vi "PosStrikerAnguloAttacker.vi"(8 "AnguloGol":dbl, 9 "atacando contra":bool, 10 "IA State":T1={"our_robots"=[], "enemy_robots"=[], "balls"=[], "geometry"={"line_width"=0, "field_length"=0, "field_width"=0, "boundary_width"=0, "referee_width"=0, "goal_width"=0, "goal_depth"=0, "goal_wall_width"=0, "center_circle_radius"=0, "defense_radius"=0, "defense_stretch"=0, "free_kick_from_defense_dist"=0, "penalty_spot_from_field_line_dist"=0, "penalty_line_from_spot_dist"=0}, "IA Judge"={"stage"="", "command"="", "our_goalie_id"=0.0, "enemy_goalie_id"=0.0, "command enum"=enum."Halt", "Time"=enum."Azul"}, "Received Timestamp"=timestamp(0 s since 1904-01-01), "Events"={"Touch"=FALSE, "Ball out"=FALSE, "id touch"=0.0, "Ball out of \nVision"=FALSE, "Ball inside \nGoalie area"=FALSE, "Robot not responding"=FALSE, "Robots responding status"=[1.0, 1.0, 1.0, 1.0, 1.0, 1.0], "Enemy Ball \nPossession"=FALSE, "Pass State"=FALSE, "id end of pass"=0.0, "Kick"=FALSE, "Id ini Possession"=0.0, "Ball Possesion"=FALSE, "Id Possesion"=0.0}}) -> (0 "YdoAttacker 2":dbl, 1 "AttackerPositive?":bool, 2 "theta final":dbl, 3 "XdoAttacker 2":dbl)   [LabVIEW 2017]
uses:
  Core/AI Input.ctl
  Core/AI Robot.ctl
  Intel/Functions Enum.ctl
  Intel/AttackerStates.ctl
  Core/AI Ball.ctl
  Core/Field Size.ctl
  Core/AI Judge.ctl
  Intel/Command Enum.ctl
  Events/Events.ctl
panel:
  in  "valor de theta 3":dbl
  in  "tamanho do intervalo 3":dbl
  in  "inicio do intervalo 3":dbl
  in  "fim do intervalo 3":dbl
  in  "Contador 4":dbl
  in  "Array 3":dbl[](array[numeric])=[0.0, 0.0, 0.0, 0.0, 0.0, 0.0]
  in  "valor de theta 2":dbl
  in  "tamanho do intervalo 2":dbl
  in  "inicio do intervalo 2":dbl
  in  "fim do intervalo 2":dbl
  in  "Contador 3":dbl
  in  "Array 2":dbl[](array[numeric])=[0.0, 0.0, 0.0, 0.0, 0.0, 0.0]
  in  "XdoAttacker":dbl
  in  "YdoAttacker":dbl
  in  "RobôsParaAnalisar":dbl[][](array[numeric])=[[99999.0, 99999.0], [99999.0, 99999.0], [99999.0, 99999.0], [99999.0, 99999.0], [99999.0, 99999.0], [99999.0, 99999.0], [99999.0, 99999.0]]
  in  "Contador":dbl
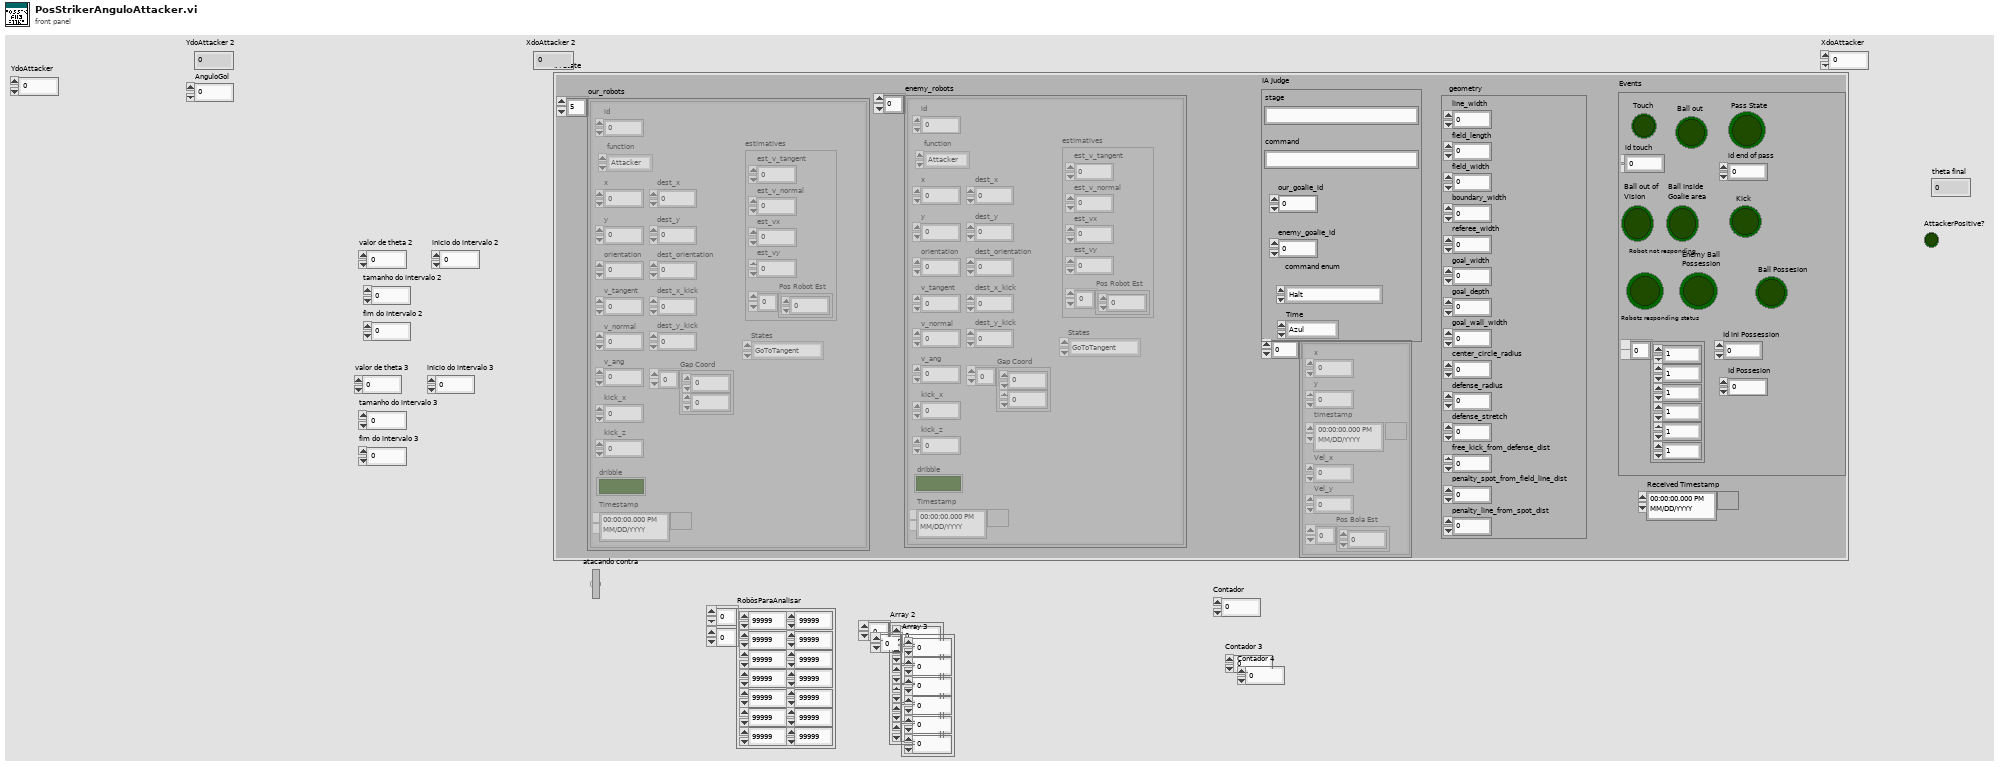
[diagram p1: front panel]
types:
  T1 = typedef "AI Input.ctl" = cluster{"our_robots":T2[], "enemy_robots":T2[], "balls":T5[], "geometry":T6, "IA Judge":T7, "Received Timestamp":timestamp, "Events":T9}
  T2 = typedef "AI Robot.ctl" = cluster{"id":u32, "function":T3, "x":dbl, "y":dbl, "orientation":dbl, "v_tangent":dbl, "v_normal":dbl, "v_ang":dbl, "kick_x":dbl, "kick_z":dbl, "dribble":bool, "Timestamp":timestamp, "dest_x":dbl, "dest_y":dbl, "dest_orientation":dbl, "estimatives":cluster{"est_v_tangent":dbl, "est_v_normal":dbl, "est_vx":dbl, "est_vy":dbl, "Pos Robot Est":dbl[]}, "dest_x_kick":dbl, "dest_y_kick":dbl, "Gap Coord":dbl[], "States":T4}
  T3 = typedef "Functions Enum.ctl" = enum16{"Attacker", "Goalie", "Defender", "Striker", "Goto 0", "Dummy", "Kicker", "ZigZag"}
  T4 = typedef "AttackerStates.ctl" = enum16{"Pass", "GoToTangent", "BallGetting", "GoToKick", ""}
  T5 = typedef "AI Ball.ctl" = cluster{"x":dbl, "y":dbl, "timestamp":timestamp, "Vel_x":dbl, "Vel_y":dbl, "Pos Bola Est":dbl[]}
  T6 = typedef "Field Size.ctl" = cluster{"line_width":u32, "field_length":u32, "field_width":u32, "boundary_width":u32, "referee_width":u32, "goal_width":u32, "goal_depth":u32, "goal_wall_width":u32, "center_circle_radius":u32, "defense_radius":u32, "defense_stretch":u32, "free_kick_from_defense_dist":u32, "penalty_spot_from_field_line_dist":u32, "penalty_line_from_spot_dist":u32}
  T7 = typedef "AI Judge.ctl" = cluster{"stage":string, "command":string, "our_goalie_id":dbl, "enemy_goalie_id":dbl, "command enum":T8, "Time":enum16{"Azul", "Amarelo"}}
  T8 = typedef "Command Enum.ctl" = enum16{"Halt", "Stop", "Force Start", "PKA Normal Start", "Prepare Kickoff Ally", "PKE Normal Start", "Prepare Kickoff Enemy", "Prepare Penalty Ally", "PPA Normal Start", "Prepare Penalty Enemy", "PPE Normal Start", "Direct Free Enemy", "Direct Free Ally", "Indirect Free Enemy", "Indirect Free Ally", "Timeout Enemy", "Timeout Ally", "Goal Enemy", "Goal Ally", "Ball Placement Enemy", "Ball Placement Ally", "Normal Half Time", "Extra Time Break", "Extra Half Time", "None", "Post Game"}
  T9 = typedef "Events.ctl" = cluster{"Touch":bool, "Ball out":bool, "id touch":dbl, "Ball out of \nVision":bool, "Ball inside \nGoalie area":bool, "Robot not responding":bool, "Robots responding status":dbl[], "Enemy Ball \nPossession":bool, "Pass State":bool, "id end of pass":dbl, "Kick":bool, "Id ini Possession":dbl, "Ball Possesion":bool, "Id Possesion":dbl}
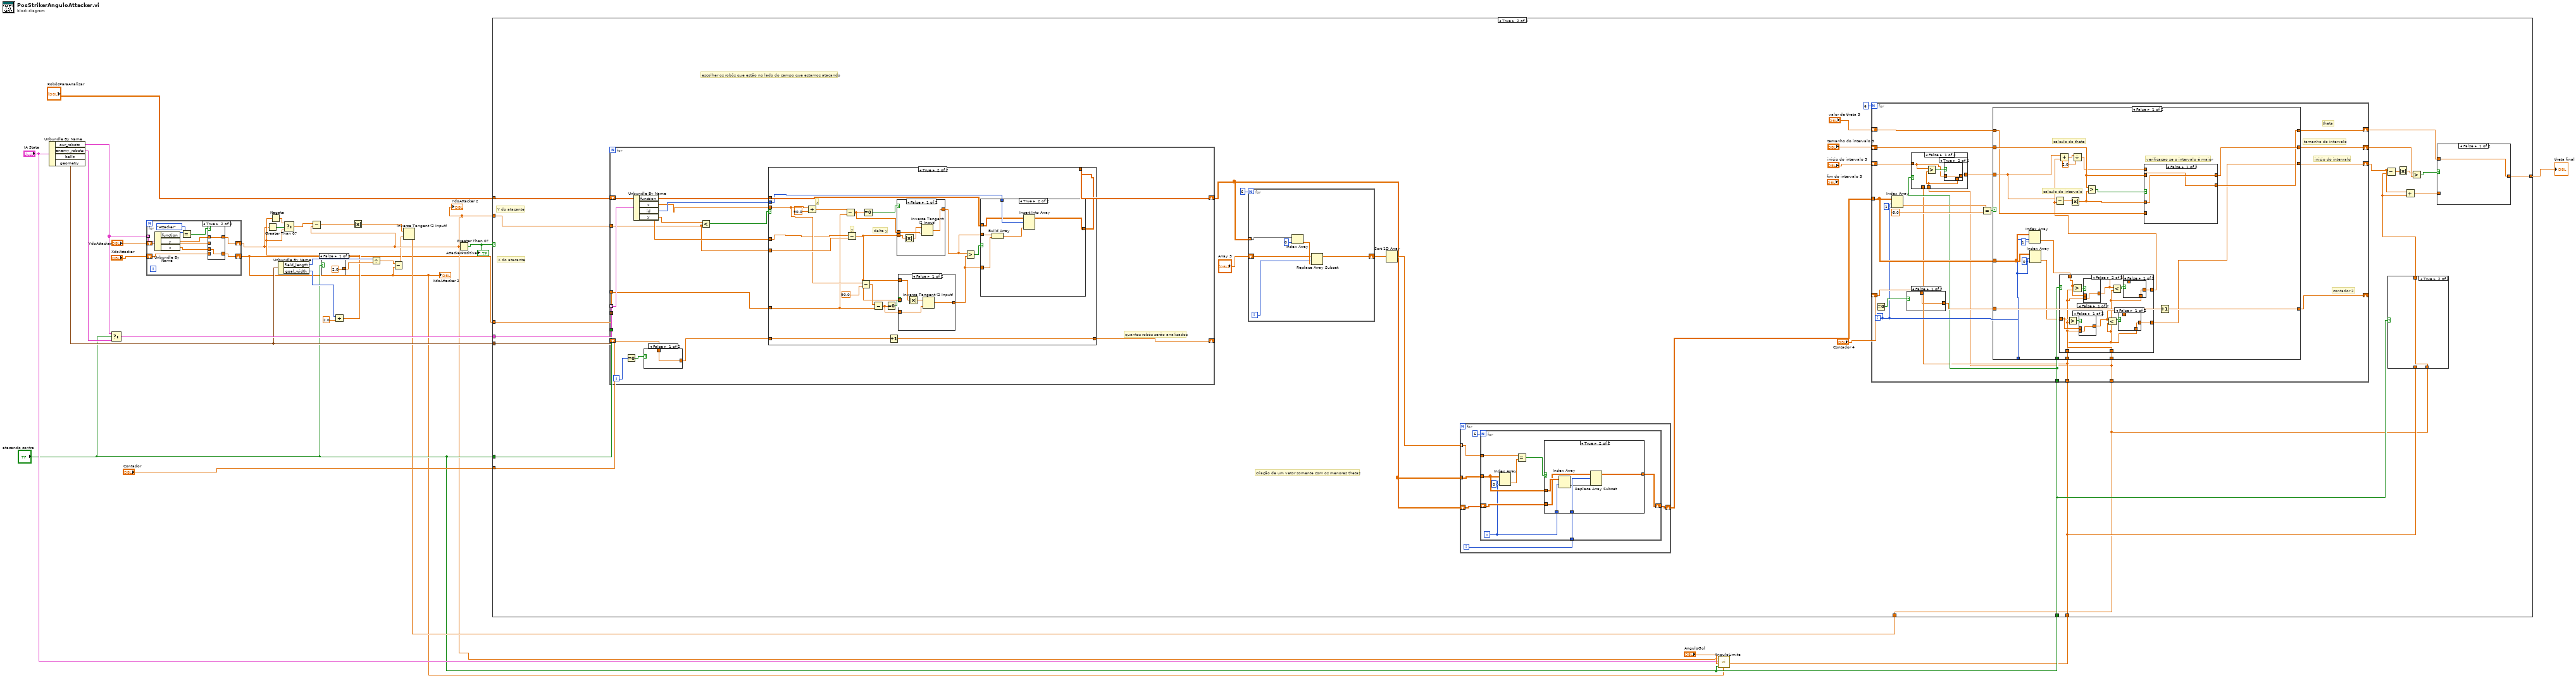
[diagram p0: block diagram]
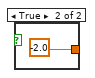
[diagram p2: hidden frame]
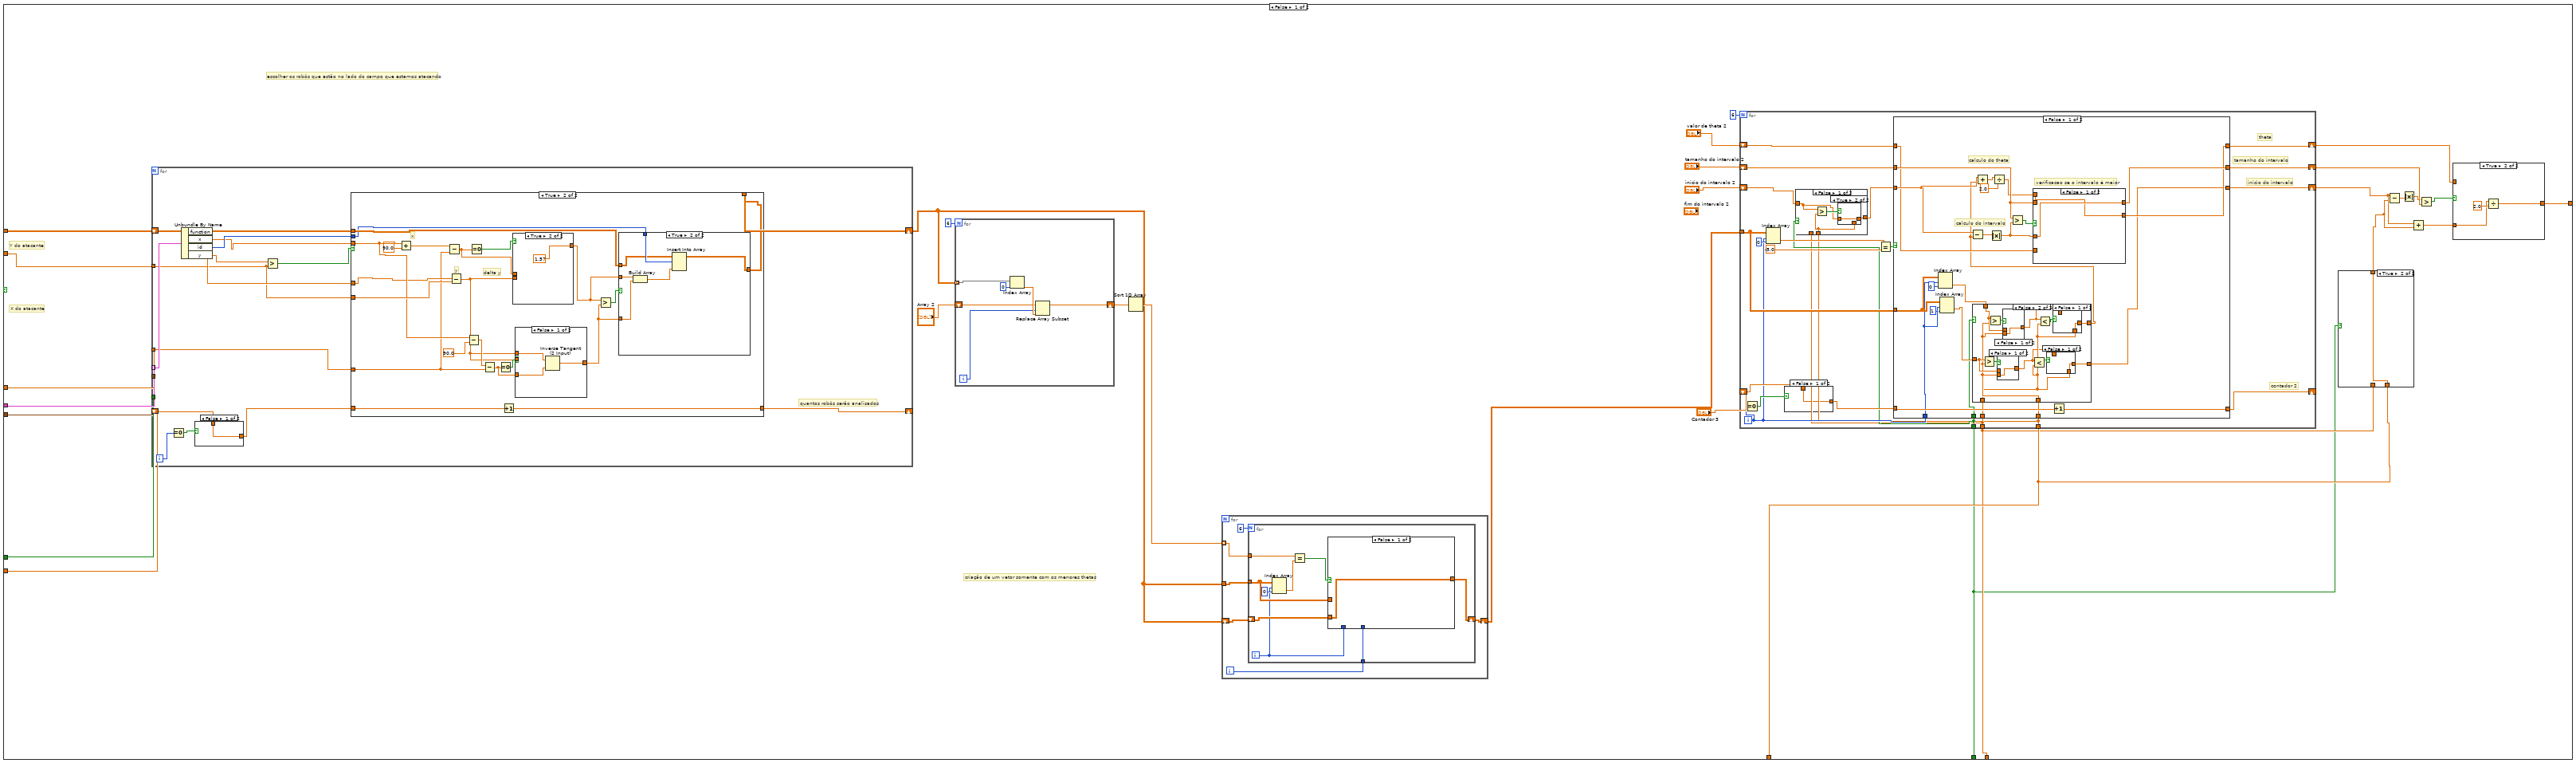
[diagram p3: hidden frame]
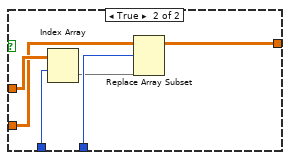
[diagram p6: hidden frame]
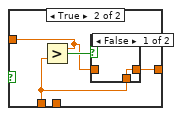
[diagram p8: hidden frame]
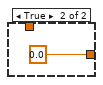
[diagram p10: hidden frame]
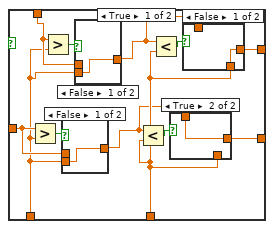
[diagram p11: hidden frame]
diagram:
  n1 = Unbundle By Name("IA State") -> ("our_robots"=w24:T2[], "enemy_robots"=w29:T2[], "geometry"=w16:T6)  [unwired: 1 out]
  n2 = Select(t=w24, s="atacando contra", f=w29) -> (s? t:f=w28:T2[])
  n3 = for {
    tunnel: w24 -> [w39] mode=indexing
    shift-right: [w34] -> w7
    shift-left: "YdoAttacker" -> [w33]
    shift-right: [w30] -> w3
    shift-left: "XdoAttacker" -> [w31]
    n4 = Unbundle By Name(w39) -> ("function"=w38:T3, "y"=w35:dbl, "x"=w32:dbl)
    n5 = Equal?(x=w38, y=Functions_Enum."Attacker") -> (x = y?=w36:bool)
    n6 = case shown="True" w36 {
      tunnel: w35 -> [_ w43]
      tunnel: [w41 w43] -> w34
      tunnel: w33 -> [w41 _]
      tunnel: w32 -> [_ w42]
      tunnel: w31 -> [w40 _]
      tunnel: [w40 w42] -> w30
      frame False {
      }
      frame True {
      }
    }
  }
  "YdoAttacker 2" <- w7
  "XdoAttacker 2" <- w3
  n7 = Greater Than 0?(x=w7) -> (x > 0?=w19:bool)
  n8 = Unbundle By Name(w16) -> ("field_length"=w20:u32, "goal_width"=w14:u32)
  n9 = case shown="False" "atacando contra" {
    tunnel: [2.0 ("y") -2.0 ("y")] -> w17
    frame False {
    }
    frame True {
    }
  }
  n10 = Divide(x=w14, y=2.0) -> (x/y=w13:dbl)
  n11 = Negate(x=w13) -> (-x=w18:dbl)
  n12 = Select(t=w18, s=w19, f=w13) -> (s? t:f=w6:dbl)
  n13 = Subtract(x=w6, y=w7) -> (x-y=w2:dbl)
  n14 = Absolute Value(x=w2) -> (abs(x)=w1:dbl)
  n15 = Divide(x=w20, y=w17) -> (x/y=w4:dbl)
  n16 = Subtract(x=w4, y=w3) -> (x-y=w5:dbl)
  n17 = Inverse Tangent (2 Input)(1:w5, 2:w1) -> (0:w12:dbl)
  n18 = Greater Than 0?(x=w7) -> (x > 0?=w21:bool)
  "AttackerPositive?" <- w21
  n19 = call "AnguloLimite.vi"("XdoAttacker"=w3, "atacando contra"="atacando contra", "AnguloGol"="AnguloGol", "IA State"="IA State", "YdoAttacker"=w7) -> ("Angulo Limite"=w8:dbl)  [unwired: 6 in]
  n20 = case shown="True" w21 {
    tunnel: w28 -> [w75 w308]
    tunnel: "atacando contra" -> [w74 w307]
    tunnel: "Contador" -> [w73 w306]
    tunnel: "RobôsParaAnalisar" -> [w72 w305]
    tunnel: w16 -> [w71 w304]
    tunnel: [w57 w290] -> w25
    tunnel: w7 -> [w51 w284]
    tunnel: w3 -> [w50 w283]
    tunnel: w12 -> [w48 w279]
    tunnel: "atacando contra" -> [w46 w282]
    tunnel: w8 -> [w47 w281]
    frame False {
      # "X do atacante"
      # "Y do atacante"
      # "criação de um vetor somente com os menores thetas"
      # "escolher os robôs que estão no lado do campo que estamos atacando"
      n21 = for {
        tunnel: w75 -> [w229] mode=indexing
        tunnel: w74 -> [_]
        shift-right: [w221] -> w61
        shift-left: w72 -> [w228]
        shift-right: [w222] -> _
        shift-left: w73 -> [w224]
        tunnel: w71 -> [_]
        tunnel: w51 -> [w217]
        tunnel: w50 -> [w216]
        i -> [w225]
        # "quantos robôs serão analisados"
        n22 = Equal To 0?(x=w225) -> (x = 0?=w226:bool)
        n23 = Unbundle By Name(w229) -> ("x"=w220:dbl, "id"=w227:u32, "y"=w219:dbl)  [unwired: 1 out]
        n24 = case shown="False" w226 {
          tunnel: w224 -> [w230 _]
          tunnel: [w230 0.0] -> w223
          frame False {
          }
          frame True {
          }
        }
        n25 = Greater?(x=w219, y=w217) -> (0:w218:bool)
        n26 = case shown="True" w218 {
          tunnel: w228 -> [w236 w256]
          tunnel: w227 -> [w235 w255]
          tunnel: w220 -> [_ w246]
          tunnel: w219 -> [_ w245]
          tunnel: w223 -> [w237 w257]
          tunnel: [w237 w258] -> w222
          tunnel: [w232 w254] -> w221
          tunnel: w217 -> [_ w247]
          tunnel: w216 -> [_ w243]
          frame False {
            w234 = -5.0 ("element")
            n27 = Build Array(w234, w234) -> (w233:dbl[])
            n28 = Insert Into Array(array=w236, index (row)=w235, new element=w233) -> (w232:dbl[][])  [unwired: 1 in]
          }
          frame True {
            # "delta y"
            # "y"
            # "x"
            n29 = Add(x=w246, y=90.0) -> (x+y=w244:dbl)
            n30 = Subtract(x=w244, y=w243) -> (x-y=w241:dbl)
            n31 = Subtract(x=w245, y=w247) -> (x-y=w238:dbl)
            n32 = Subtract(x=w246, y=90.0) -> (x-y=w251:dbl)
            n33 = Equal To 0?(x=w241) -> (x = 0?=w242:bool)
            n34 = Subtract(x=w251, y=w243) -> (x-y=w239:dbl)
            n35 = Equal To 0?(x=w239) -> (x = 0?=w240:bool)
            n36 = Increment(x=w257) -> (x+1=w258:dbl)
            n37 = case shown="True" w242 {
              tunnel: [w276 1.57] -> w249
              tunnel: w238 -> [w277 _]
              tunnel: w241 -> [w275 _]
              frame False {
                n38 = Inverse Tangent (2 Input)(1:w275, 2:w277) -> (0:w276:dbl)
              }
              frame True {
              }
            }
            n39 = case shown="False" w240 {
              tunnel: [w261 1.57] -> w248
              tunnel: w238 -> [_ _]
              tunnel: w239 -> [w260 _]
              tunnel: w238 -> [w259 _]
              frame False {
                n40 = Inverse Tangent (2 Input)(1:w260, 2:w259) -> (0:w261:dbl)
              }
              frame True {
              }
            }
            n41 = Greater?(x=w249, y=w248) -> (0:w250:bool)
            n42 = case shown="True" w250 {
              tunnel: w256 -> [w265 w271]
              tunnel: w255 -> [w267 w274]
              tunnel: w249 -> [w264 w272]
              tunnel: w248 -> [w266 w270]
              tunnel: [w263 w269] -> w254
              frame False {
                n43 = Build Array(w266, w264) -> (w268:dbl[])
                n44 = Insert Into Array(array=w265, index (row)=w267, new element=w268) -> (w263:dbl[][])  [unwired: 1 in]
              }
              frame True {
                n45 = Build Array(w272, w270) -> (w273:dbl[])
                n46 = Insert Into Array(array=w271, index (row)=w274, new element=w273) -> (w269:dbl[][])  [unwired: 1 in]
              }
            }
          }
        }
      }
      n47 = for {
        N: 6 -> [_]
        tunnel: w61 -> [w109] mode=indexing
        shift-right: [w104] -> w63
        shift-left: "Array 2" -> [w105]
        i -> [w106]
        n48 = Index Array(array=w109, index=0) -> (element=w107:dbl)
        n49 = Replace Array Subset(array=w105, new element=w107, index=w106) -> (w104:dbl[])
      }
      n50 = Sort 1D Array(array=w63) -> (sorted array=w62:dbl[])
      n51 = for {
        tunnel: w62 -> [w84] mode=indexing
        tunnel: w61 -> [w86]
        shift-right: [w82] -> w60
        shift-left: w61 -> [w85]
        i -> [w83]
        n52 = for {
          N: 6 -> [_]
          tunnel: w86 -> [w92]
          shift-right: [w88] -> w82
          shift-left: w85 -> [w91]
          tunnel: w84 -> [w94]
          tunnel: w83 -> [w89]
          i -> [w90]
          n53 = Index Array(array=w92, index (row)=w90, index (col)=0 ("disabled index (col)")) -> (element=w95:dbl)
          n54 = Equal?(x=w94, y=w95) -> (x = y?=w93:bool)
          n55 = case shown="False" w93 {
            tunnel: w92 -> [_ w103]
            tunnel: w91 -> [w97 w99]
            tunnel: w90 -> [_ w102]
            tunnel: w89 -> [_ w101]
            tunnel: [w97 w98] -> w88
            frame False {
            }
            frame True {
              n56 = Index Array(array=w103, index (row)=w102) -> (element=w100:dbl[])  [unwired: 1 in]
              n57 = Replace Array Subset(array=w99, new element=w100, index (row)=w101) -> (w98:dbl[][])  [unwired: 1 in]
            }
          }
        }
      }
      n58 = for {
        N: 6 -> [_]
        tunnel: w60 -> [w116]
        shift-right: [w124] -> w56
        shift-left: "valor de theta 2" -> [w125]
        shift-right: [w122] -> w59
        shift-left: "tamanho do intervalo 2" -> [w123]
        shift-right: [w121] -> w53
        shift-left: "inicio do intervalo 2" -> [w113]
        shift-right: [w117] -> _
        shift-left: "Contador 3" -> [w119]
        tunnel: w47 -> [w111]
        tunnel: w48 -> [w110]
        tunnel: w46 -> [w114]
        i -> [w115]
        # "contador 2"
        # "inicio do intervalo"
        # "tamanho do intervalo"
        # "theta"
        n59 = Equal To 0?(x=w115) -> (x = 0?=w120:bool)
        n60 = Index Array(array=w116, index (row)=w115, index (col)=0 ("disabled index (col)")) -> (element=w127:dbl)
        n61 = case shown="False" w120 {
          tunnel: w119 -> [w142 _]
          tunnel: [w142 0.0] -> w118
          frame False {
          }
          frame True {
          }
        }
        n62 = case shown="False" w114 {
          tunnel: w111 -> [_ w136]
          tunnel: w113 -> [w132 w137]
          tunnel: [w130 w138] -> w112
          tunnel: w110 -> [w131 _]
          frame False {
            n63 = Greater?(x=w132, y=w131) -> (0:w133:bool)
            n64 = case shown="True" w133 {
              tunnel: [w134 w135] -> w130
              tunnel: w132 -> [_ w135]
              tunnel: w131 -> [w134 _]
              frame False {
              }
              frame True {
              }
            }
          }
          frame True {
            n65 = Greater?(x=w137, y=w136) -> (0:w139:bool)
            n66 = case shown="False" w139 {
              tunnel: [w140 w141] -> w138
              tunnel: w137 -> [_ w141]
              tunnel: w136 -> [w140 _]
              frame False {
              }
              frame True {
              }
            }
          }
        }
        n67 = Equal?(x=w127, y=-5.0) -> (x = y?=w128:bool)
        n68 = case shown="False" w128 {
          tunnel: w125 -> [w151 w215]
          tunnel: [w152 w215] -> w124
          tunnel: w123 -> [w156 w214]
          tunnel: [w155 w214] -> w122
          tunnel: w112 -> [w167 w213]
          tunnel: [w149 w213] -> w121
          tunnel: w118 -> [w165 w212]
          tunnel: [w166 w212] -> w117
          tunnel: w116 -> [w164 _]
          tunnel: w115 -> [w163 _]
          tunnel: w111 -> [w146 _]
          tunnel: w110 -> [w145 _]
          tunnel: w114 -> [w144 _]
          frame False {
            # "calculo do theta"
            # "calculo do intervalo"
            # "verificacao se o intervalo é maior"
            n69 = Index Array(array=w164, index (row)=w163, index (col)=0 ("disabled index (col)")) -> (element=w148:dbl)
            n70 = Index Array(array=w164, index (row)=w163, index (col)=1 ("disabled index (col)")) -> (element=w150:dbl)
            n71 = case shown="False" w144 {
              tunnel: w146 -> [w171 w189]
              tunnel: w148 -> [w178 w198]
              tunnel: w145 -> [w170 w190]
              tunnel: [w176 w196] -> w147
              tunnel: w150 -> [w172 w192]
              tunnel: [w169 w191] -> w149
              frame True {
                n72 = Greater?(x=w172, y=w171) -> (0:w174:bool)
                n73 = Greater?(x=w178, y=w171) -> (0:w179:bool)
                n74 = case shown="False" w174 {
                  tunnel: [w182 w183] -> w168
                  tunnel: w172 -> [_ w183]
                  tunnel: w171 -> [w182 _]
                  frame False {
                  }
                  frame True {
                  }
                }
                n75 = case shown="False" w179 {
                  tunnel: [w186 w187] -> w175
                  tunnel: w178 -> [_ w187]
                  tunnel: w171 -> [w186 _]
                  frame False {
                  }
                  frame True {
                  }
                }
                n76 = Less?(x=w168, y=w170) -> (x < y?=w173:bool)
                n77 = Less?(x=w175, y=w170) -> (x < y?=w177:bool)
                n78 = case shown="True" w173 {
                  tunnel: [w180 w181] -> w169
                  tunnel: w168 -> [_ w181]
                  tunnel: w170 -> [w180 _]
                  frame False {
                  }
                  frame True {
                  }
                }
                n79 = case shown="False" w177 {
                  tunnel: [w184 w185] -> w176
                  tunnel: w175 -> [_ w185]
                  tunnel: w170 -> [w184 _]
                  frame False {
                  }
                  frame True {
                  }
                }
              }
              frame False {
                n80 = Greater?(x=w192, y=w190) -> (0:w194:bool)
                n81 = Greater?(x=w198, y=w190) -> (0:w199:bool)
                n82 = case shown="False" w194 {
                  tunnel: [w202 w203] -> w188
                  tunnel: w192 -> [_ w203]
                  tunnel: w190 -> [w202 _]
                  frame False {
                  }
                  frame True {
                  }
                }
                n83 = case shown="False" w199 {
                  tunnel: [w206 w207] -> w195
                  tunnel: w198 -> [_ w207]
                  tunnel: w190 -> [w206 _]
                  frame False {
                  }
                  frame True {
                  }
                }
                n84 = Less?(x=w188, y=w189) -> (x < y?=w193:bool)
                n85 = Less?(x=w195, y=w189) -> (x < y?=w197:bool)
                n86 = case shown="False" w193 {
                  tunnel: [w200 w201] -> w191
                  tunnel: w188 -> [_ w201]
                  tunnel: w189 -> [w200 _]
                  frame False {
                  }
                  frame True {
                  }
                }
                n87 = case shown="False" w197 {
                  tunnel: [w204 w205] -> w196
                  tunnel: w195 -> [_ w205]
                  tunnel: w189 -> [w204 _]
                  frame False {
                  }
                  frame True {
                  }
                }
              }
            }
            n88 = Subtract(x=w167, y=w147) -> (x-y=w160:dbl)
            n89 = Add(x=w167, y=w147) -> (x+y=w159:dbl)
            n90 = Absolute Value(x=w160) -> (abs(x)=w154:dbl)
            n91 = Divide(x=w159, y=2.0) -> (x/y=w153:dbl)
            n92 = Greater?(x=w156, y=w154) -> (0:w157:bool)
            n93 = case shown="False" w157 {
              tunnel: w156 -> [_ w211]
              tunnel: [w209 w211] -> w155
              tunnel: w154 -> [w209 _]
              tunnel: w151 -> [_ w210]
              tunnel: w153 -> [w208 _]
              tunnel: [w208 w210] -> w152
              frame False {
              }
              frame True {
              }
            }
            n94 = Increment(x=w165) -> (x+1=w166:dbl)
          }
          frame True {
          }
        }
      }
      n95 = case shown="True" w46 {
        tunnel: w47 -> [w76 _]
        tunnel: [w76 w77] -> w49
        tunnel: w48 -> [_ w77]
        frame False {
        }
        frame True {
        }
      }
      n96 = Subtract(x=w53, y=w49) -> (x-y=w55:dbl)
      n97 = Absolute Value(x=w55) -> (abs(x)=w54:dbl)
      n98 = Add(x=w53, y=w49) -> (x+y=w52:dbl)
      n99 = Greater?(x=w54, y=w59) -> (0:w58:bool)
      n100 = case shown="True" w58 {
        tunnel: [w78 w80] -> w57
        tunnel: w56 -> [w78 _]
        tunnel: w52 -> [_ w79]
        frame False {
        }
        frame True {
          n101 = Divide(x=w79, y=2.0) -> (x/y=w80:dbl)
        }
      }
    }
    frame True {
      # "X do atacante"
      # "Y do atacante"
      # "criação de um vetor somente com os menores thetas"
      # "escolher os robôs que estão no lado do campo que estamos atacando"
      n102 = for {
        tunnel: w308 -> [w462] mode=indexing
        tunnel: w307 -> [_]
        shift-right: [w454] -> w294
        shift-left: w305 -> [w461]
        shift-right: [w455] -> _
        shift-left: w306 -> [w457]
        tunnel: w304 -> [_]
        tunnel: w284 -> [w450]
        tunnel: w283 -> [w449]
        i -> [w458]
        # "quantos robôs serão analisados"
        n103 = Equal To 0?(x=w458) -> (x = 0?=w459:bool)
        n104 = Unbundle By Name(w462) -> ("x"=w453:dbl, "id"=w460:u32, "y"=w452:dbl)  [unwired: 1 out]
        n105 = case shown="False" w459 {
          tunnel: w457 -> [w463 _]
          tunnel: [w463 0.0] -> w456
          frame False {
          }
          frame True {
          }
        }
        n106 = Less?(x=w452, y=w450) -> (x < y?=w451:bool)
        n107 = case shown="True" w451 {
          tunnel: w461 -> [w469 w489]
          tunnel: w460 -> [w468 w488]
          tunnel: w453 -> [_ w479]
          tunnel: w452 -> [_ w478]
          tunnel: w456 -> [w470 w490]
          tunnel: [w470 w491] -> w455
          tunnel: [w465 w487] -> w454
          tunnel: w450 -> [_ w480]
          tunnel: w449 -> [_ w476]
          frame False {
            w467 = -5.0 ("element")
            n108 = Build Array(w467, w467) -> (w466:dbl[])
            n109 = Insert Into Array(array=w469, index (row)=w468, new element=w466) -> (w465:dbl[][])  [unwired: 1 in]
          }
          frame True {
            # "delta y"
            # "y"
            # "x"
            n110 = Add(x=w479, y=90.0) -> (x+y=w477:dbl)
            n111 = Subtract(x=w477, y=w476) -> (x-y=w474:dbl)
            n112 = Subtract(x=w478, y=w480) -> (x-y=w471:dbl)
            n113 = Subtract(x=w479, y=90.0) -> (x-y=w484:dbl)
            n114 = Equal To 0?(x=w474) -> (x = 0?=w475:bool)
            n115 = Subtract(x=w484, y=w476) -> (x-y=w472:dbl)
            n116 = Equal To 0?(x=w472) -> (x = 0?=w473:bool)
            n117 = Increment(x=w490) -> (x+1=w491:dbl)
            n118 = case shown="False" w475 {
              tunnel: [w512 1.57] -> w482
              tunnel: w471 -> [w510 _]
              tunnel: w474 -> [w511 _]
              frame False {
                n119 = Absolute Value(x=w510) -> (abs(x)=w509:dbl)
                n120 = Inverse Tangent (2 Input)(1:w511, 2:w509) -> (0:w512:dbl)
              }
              frame True {
              }
            }
            n121 = case shown="False" w473 {
              tunnel: [w495 1.57] -> w481
              tunnel: w471 -> [_ _]
              tunnel: w472 -> [w494 _]
              tunnel: w471 -> [w492 _]
              frame False {
                n122 = Absolute Value(x=w492) -> (abs(x)=w493:dbl)
                n123 = Inverse Tangent (2 Input)(1:w494, 2:w493) -> (0:w495:dbl)
              }
              frame True {
              }
            }
            n124 = Greater?(x=w482, y=w481) -> (0:w483:bool)
            n125 = case shown="True" w483 {
              tunnel: w489 -> [w499 w505]
              tunnel: w488 -> [w501 w508]
              tunnel: w482 -> [w498 w506]
              tunnel: w481 -> [w500 w504]
              tunnel: [w497 w503] -> w487
              frame False {
                n126 = Build Array(w500, w498) -> (w502:dbl[])
                n127 = Insert Into Array(array=w499, index (row)=w501, new element=w502) -> (w497:dbl[][])  [unwired: 1 in]
              }
              frame True {
                n128 = Build Array(w506, w504) -> (w507:dbl[])
                n129 = Insert Into Array(array=w505, index (row)=w508, new element=w507) -> (w503:dbl[][])  [unwired: 1 in]
              }
            }
          }
        }
      }
      n130 = for {
        N: 6 -> [_]
        tunnel: w294 -> [w342] mode=indexing
        shift-right: [w337] -> w296
        shift-left: "Array 3" -> [w338]
        i -> [w339]
        n131 = Index Array(array=w342, index=0) -> (element=w340:dbl)
        n132 = Replace Array Subset(array=w338, new element=w340, index=w339) -> (w337:dbl[])
      }
      n133 = Sort 1D Array(array=w296) -> (sorted array=w295:dbl[])
      n134 = for {
        tunnel: w295 -> [w317] mode=indexing
        tunnel: w294 -> [w319]
        shift-right: [w315] -> w293
        shift-left: w294 -> [w318]
        i -> [w316]
        n135 = for {
          N: 6 -> [_]
          tunnel: w319 -> [w325]
          shift-right: [w321] -> w315
          shift-left: w318 -> [w324]
          tunnel: w317 -> [w327]
          tunnel: w316 -> [w322]
          i -> [w323]
          n136 = Index Array(array=w325, index (row)=w323, index (col)=0 ("disabled index (col)")) -> (element=w328:dbl)
          n137 = Equal?(x=w327, y=w328) -> (x = y?=w326:bool)
          n138 = case shown="True" w326 {
            tunnel: w325 -> [_ w336]
            tunnel: w324 -> [w330 w332]
            tunnel: w323 -> [_ w335]
            tunnel: w322 -> [_ w334]
            tunnel: [w330 w331] -> w321
            frame False {
            }
            frame True {
              n139 = Index Array(array=w336, index (row)=w335) -> (element=w333:dbl[])  [unwired: 1 in]
              n140 = Replace Array Subset(array=w332, new element=w333, index (row)=w334) -> (w331:dbl[][])  [unwired: 1 in]
            }
          }
        }
      }
      n141 = for {
        N: 6 -> [_]
        tunnel: w293 -> [w349]
        shift-right: [w357] -> w289
        shift-left: "valor de theta 3" -> [w358]
        shift-right: [w355] -> w292
        shift-left: "tamanho do intervalo 3" -> [w356]
        shift-right: [w354] -> w286
        shift-left: "inicio do intervalo 3" -> [w345]
        shift-right: [w350] -> _
        shift-left: "Contador 4" -> [w352]
        tunnel: w282 -> [w347]
        tunnel: w281 -> [w346]
        tunnel: w279 -> [w343]
        i -> [w348]
        # "contador 2"
        # "inicio do intervalo"
        # "tamanho do intervalo"
        # "theta"
        n142 = Equal To 0?(x=w348) -> (x = 0?=w353:bool)
        n143 = Index Array(array=w349, index (row)=w348, index (col)=1 ("disabled index (col)")) -> (element=w360:dbl)
        n144 = case shown="False" w353 {
          tunnel: w352 -> [w375 _]
          tunnel: [w375 0.0] -> w351
          frame False {
          }
          frame True {
          }
        }
        n145 = case shown="False" w347 {
          tunnel: w346 -> [_ w369]
          tunnel: w345 -> [w365 w370]
          tunnel: [w363 w371] -> w344
          tunnel: w343 -> [w364 _]
          frame False {
            n146 = Greater?(x=w365, y=w364) -> (0:w366:bool)
            n147 = case shown="True" w366 {
              tunnel: [w367 w368] -> w363
              tunnel: w365 -> [_ w368]
              tunnel: w364 -> [w367 _]
              frame False {
              }
              frame True {
              }
            }
          }
          frame True {
            n148 = Greater?(x=w370, y=w369) -> (0:w372:bool)
            n149 = case shown="False" w372 {
              tunnel: [w373 w374] -> w371
              tunnel: w370 -> [_ w374]
              tunnel: w369 -> [w373 _]
              frame False {
              }
              frame True {
              }
            }
          }
        }
        n150 = Equal?(x=w360, y=-5.0) -> (x = y?=w361:bool)
        n151 = case shown="False" w361 {
          tunnel: w358 -> [w385 w448]
          tunnel: [w386 w448] -> w357
          tunnel: w356 -> [w390 w447]
          tunnel: [w389 w447] -> w355
          tunnel: [w379 w445] -> w354
          tunnel: w351 -> [w399 w446]
          tunnel: [w400 w446] -> w350
          tunnel: w349 -> [w398 _]
          tunnel: w348 -> [w397 _]
          tunnel: w347 -> [w384 _]
          tunnel: w346 -> [w383 _]
          tunnel: w343 -> [w382 _]
          tunnel: w344 -> [w378 w445]
          frame False {
            # "calculo do theta"
            # "calculo do intervalo"
            # "verificacao se o intervalo é maior"
            n152 = Index Array(array=w398, index (row)=w397, index (col)=1 ("disabled index (col)")) -> (element=w377:dbl)
            n153 = Index Array(array=w398, index (row)=w397, index (col)=0 ("disabled index (col)")) -> (element=w380:dbl)
            n154 = case shown="False" w384 {
              tunnel: w383 -> [w404 w422]
              tunnel: w377 -> [w411 w431]
              tunnel: w382 -> [w403 w423]
              tunnel: [w409 w429] -> w381
              tunnel: w380 -> [w405 w425]
              tunnel: [w402 w424] -> w379
              frame True {
                n155 = Greater?(x=w405, y=w404) -> (0:w407:bool)
                n156 = Greater?(x=w411, y=w404) -> (0:w412:bool)
                n157 = case shown="False" w407 {
                  tunnel: [w415 w416] -> w401
                  tunnel: w405 -> [_ w416]
                  tunnel: w404 -> [w415 _]
                  frame False {
                  }
                  frame True {
                  }
                }
                n158 = case shown="False" w412 {
                  tunnel: [w419 w420] -> w408
                  tunnel: w411 -> [_ w420]
                  tunnel: w404 -> [w419 _]
                  frame False {
                  }
                  frame True {
                  }
                }
                n159 = Less?(x=w401, y=w403) -> (x < y?=w406:bool)
                n160 = Less?(x=w408, y=w403) -> (x < y?=w410:bool)
                n161 = case shown="True" w406 {
                  tunnel: [w413 w414] -> w402
                  tunnel: w401 -> [_ w414]
                  tunnel: w403 -> [w413 _]
                  frame False {
                  }
                  frame True {
                  }
                }
                n162 = case shown="False" w410 {
                  tunnel: [w417 w418] -> w409
                  tunnel: w408 -> [_ w418]
                  tunnel: w403 -> [w417 _]
                  frame False {
                  }
                  frame True {
                  }
                }
              }
              frame False {
                n163 = Greater?(x=w425, y=w423) -> (0:w427:bool)
                n164 = Greater?(x=w431, y=w423) -> (0:w432:bool)
                n165 = case shown="False" w427 {
                  tunnel: [w435 w436] -> w421
                  tunnel: w425 -> [_ w436]
                  tunnel: w423 -> [w435 _]
                  frame False {
                  }
                  frame True {
                  }
                }
                n166 = case shown="False" w432 {
                  tunnel: [w439 w440] -> w428
                  tunnel: w431 -> [_ w440]
                  tunnel: w423 -> [w439 _]
                  frame False {
                  }
                  frame True {
                  }
                }
                n167 = Less?(x=w421, y=w422) -> (x < y?=w426:bool)
                n168 = Less?(x=w428, y=w422) -> (x < y?=w430:bool)
                n169 = case shown="False" w426 {
                  tunnel: [w433 w434] -> w424
                  tunnel: w421 -> [_ w434]
                  tunnel: w422 -> [w433 _]
                  frame False {
                  }
                  frame True {
                  }
                }
                n170 = case shown="False" w430 {
                  tunnel: [w437 w438] -> w429
                  tunnel: w428 -> [_ w438]
                  tunnel: w422 -> [w437 _]
                  frame False {
                  }
                  frame True {
                  }
                }
              }
            }
            n171 = Subtract(x=w378, y=w381) -> (x-y=w394:dbl)
            n172 = Add(x=w378, y=w381) -> (x+y=w393:dbl)
            n173 = Absolute Value(x=w394) -> (abs(x)=w388:dbl)
            n174 = Divide(x=w393, y=2.0) -> (x/y=w387:dbl)
            n175 = Greater?(x=w390, y=w388) -> (0:w391:bool)
            n176 = case shown="False" w391 {
              tunnel: w390 -> [_ w444]
              tunnel: [w442 w444] -> w389
              tunnel: w388 -> [w442 _]
              tunnel: w385 -> [_ w443]
              tunnel: w387 -> [w441 _]
              tunnel: [w441 w443] -> w386
              frame False {
              }
              frame True {
              }
            }
            n177 = Increment(x=w399) -> (x+1=w400:dbl)
          }
          frame True {
          }
        }
      }
      n178 = case shown="True" w282 {
        tunnel: w281 -> [w309 _]
        tunnel: [w309 w310] -> w280
        tunnel: w279 -> [_ w310]
        frame False {
        }
        frame True {
        }
      }
      n179 = Subtract(x=w286, y=w280) -> (x-y=w288:dbl)
      n180 = Absolute Value(x=w288) -> (abs(x)=w287:dbl)
      n181 = Add(x=w286, y=w280) -> (x+y=w285:dbl)
      n182 = Greater?(x=w287, y=w292) -> (0:w291:bool)
      n183 = case shown="False" w291 {
        tunnel: [w311 w313] -> w290
        tunnel: w289 -> [w311 _]
        tunnel: w285 -> [_ w312]
        frame False {
        }
        frame True {
          n184 = Divide(x=w312, y=2.0) -> (x/y=w313:dbl)
        }
      }
    }
  }
  "theta final" <- w25
